vi "H-Bridge Motor Testing.vi"() -> ()   [LabVIEW 2025]
uses:
  <vilib>/MakerHub/LINX/Public/Utilities/Open Serial.vi
  <vilib>/MakerHub/LINX/Public/Peripherals/PWM/PWM Set Duty Cycle N Chans.vi
  <vilib>/MakerHub/LINX/LMH-LINX.lvlib
panel:
  in  "-":dbl
  in  "+":dbl
  in  "IN 4":i32
  in  "IN 3":i32
  in  "IN 2":i32
  in  "- 2":dbl
  in  "IN 1":i32 min=0 max=13 step=1
  in  "+ 2":dbl
  in  "Serial Port":refnum<visa-resource-name>="N/A"
  in  "?":bool
  # "This is a test program used to verify the operation of the H-Bridge and to visually demonstrate the functioning of PWM, using the Arduino as a microcontroller. The program was developed at the Applied Control Laboratory (LCA) of the Federal Institute of São Paulo by students Guilherme Tinoco and Eduardo Piassi."
  # "PWM MOTOR 1"
  # "PWM MOTOR 2"
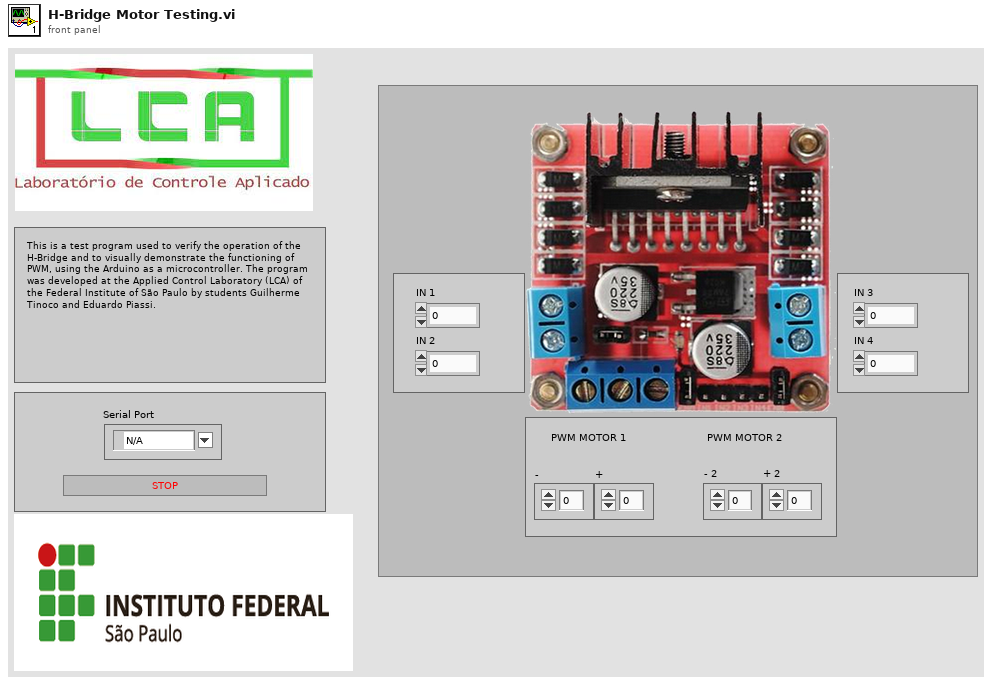
[diagram p1: front panel]
types:
  T1 = typedef "LMH-LINX.lvlib/LINX Ref.ctl" = cluster{"IO":T2, "Interface":T3, "LINX Device Config":T4}
  T2 = typedef "LMH-LINX.lvlib/Platform.ctl" = enum16{"Remote", "Local"}
  T3 = typedef "LMH-LINX.lvlib/Interface.ctl" = enum16{"Serial", "TCP"}
  T4 = typedef "LMH-LINX.lvlib/Device.lvlib/LINX Device Config.ctl" = cluster{"Interface":T3, "COM Port":refnum<visa-resource-name>, "TCP Configuration":T5, "Device Family":u8, "Device ID":u8, "Device Name":string, "TCP Ref":refnum<k5>, "Channels":T6}
  T5 = typedef "LMH-LINX.lvlib/Device.lvlib/TCP Config.ctl" = cluster{"IP Address":string, "Port":u16}
  T6 = typedef "LMH-LINX.lvlib/Channels.ctl" = cluster{"DI":u8[], "DO":u8[], "AI":u8[], "AO":u8[], "PWM":u8[], "QE":u8[], "UART":u8[], "I2C 2":u8[], "SPI":u8[], "CAN":u8[], "Servo":u8[], "AI Ref (V)":dbl, "AI Resolution (Bits)":u8, "AO Ref (V)":dbl, "AO Resolution (Bits)":u8}
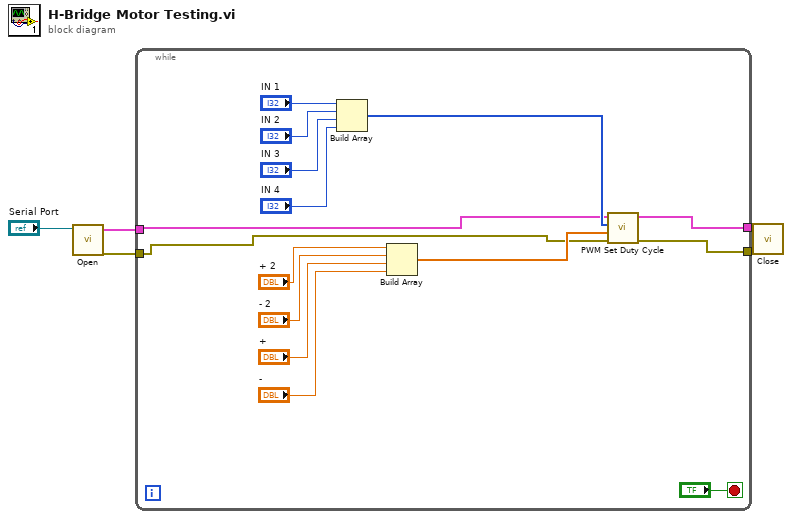
[diagram p0: block diagram]
diagram:
  n1 = call-poly <vilib>:"Open.vi"("Serial Port"="Serial Port") -> ("Error Out"=w4:errorcluster, "LINX Resource"=w5:T1)  [unwired: 8 in, 1 out]
  n2 = while {
    tunnel: w5 -> [w6]
    tunnel: w4 -> [w7]
    tunnel: [w9] -> w3
    tunnel: [w8] -> w2
    stop <- "?" stop-if-true
    n3 = Build Array("IN 1", "IN 2", "IN 3", "IN 4") -> (w18:i32[])
    n4 = Build Array("+ 2", "- 2", "+", "-") -> (w10:dbl[])
    n5 = call-poly <vilib>:"PWM Set Duty Cycle.vi"("Error In"=w7, "Duty Cycles"=w10, "PWM Channels"=w18, "LINX Resource"=w6) -> ("Error Out"=w8:errorcluster, "LINX Resource"=w9:T1)  [unwired: 6 in]
  }
  n6 = call <vilib>:"Close.vi"("Error In"=w2, "LINX Resource"=w3) -> ()  [unwired: 9 in, 1 out]
